vi "force_ctrl_test.vi"() -> ()   [LabVIEW 2014]
uses:
  <vilib>/eio/EIONode/EIONode.xnode
  <vilib>/rvi/FXPMathLib/FxpMul/XNode/nifxpmath_Multiplier.xnode
  <vilib>/rvi/FXPMathLib/sim/FxpSim.dll
  <vilib>/rvi/eio/common/nirviEmuTemplateMethod_errors.vi
  <vilib>/rvi/FXPMathLib/FxpSinAndCos/XNode/nifxpmath_SinAndCos.xnode
  <vilib>/rvi/FXPMathLib/FxpSinAndCos/simVIs/DllFxpSinAndCosTemp_sub.vi
  <vilib>/rvi/FXPMathLib/FxpSinAndCos/subVIs/nifxpmath_SinAndCos_SimConfig.ctl
  <vilib>/rvi/Analysis/measure/butterworth/XNode/niFpgaButterworthFilter.xnode
  <vilib>/rvi/FXPMathLib/FxpSub/XNode/nifxpmath_Sub.xnode
  <vilib>/rvi/FXPMathLib/FxpAdd/XNode/nifxpmath_Add.xnode
  <vilib>/rvi/DataTransferAndStorage/Container/XNode/niFpgaContainer.xnode
  <vilib>/rvi/interface/RandomDataEmulation/nirviRandomDataFpgaMultiElementTemplate.vi
panel:
  out "Mod6/AI0":fxp<+/-,24,-4>
  out "Chirp Frequency (Hz)":fxp<+/-,30,7>
  in  "Frequency_start (Hz)":fxp<+/-,36,4>
  in  "Target time (s)":fxp<+/-,36,11>
  in  "Frequency_end (Hz)":fxp<+/-,33,6>
  out "Chirp_signal":fxp<+/-,36,11>
  in  "Sin wave ampitude (mm)":fxp<+/-,33,6>
  out "omega (M_avg)":fxp<+/-,64,35>
  out "D_d (M_avg)":fxp<+/-,64,32>
  in  "D_d_M_avg_Tc (uSec)":u32
  out "omega (M)":fxp<+/-,64,30>
  out "D_d (M)":fxp<+/-,64,27>
  in  "D_d_M_Tc (uSec)":u32 format="%#_6f"
  out "D_d (T)":fxp<+/-,46,10>
  out "omega(T)":fxp<+/-,20,9>
  in  "Velocity Estimation":i16(ring) items=["M_avg method", "M method", "T method"]
  out "Dr_ramp":fxp<+/-,64,30>
  out "Dr_slope":fxp<+/-,33,17>
  in  "Dr_time":fxp<+/-,16,11>
  out "Dr_sin":fxp<+/-,28,11>
  out "Dr_sin_d":fxp<+/-,64,16>
  out "Dr_sin_dd":fxp<+/-,64,25>
  out "Sin omega":fxp<+/-,41,8>
  in  "Sin offset":fxp<+/-,27,10>
  in  "Sin magnitude":fxp<+/-,11,8>
  in  "Sin wave frequency (Hz)":fxp<+/-,21,5>
  out "Time now (s)":fxp<+,52,14>
  out "Dr":fxp<+/-,64,31>
  in  "Dr_end":fxp<+/-,16,11>
  in  "Command type":i16(ring) items=["Step", "Ramp", "Sine", "Chirp"]
  out "D_i":fxp<+/-,38,10>
  in  "D_tolorence":fxp<+/-,27,3>
  in  "Ki":fxp<+/-,36,10>
  out "D_error":fxp<+/-,36,10>
  in  "Direction":bool
  out "Fmr_PD":fxp<+/-,36,10>
  in  "Kd":fxp<+/-,36,10>
  in  "Kp":fxp<+/-,33,10>
  in  "scaled coefficients_D_dd":i32[](array[numeric])=[780119100, 146811362]
  out "D_dd":fxp<+/-,36,29>
  in  "Ini coe.":bool
  out "va":fxp<+/-,43,8>
  out "vb":fxp<+/-,43,8>
  in  "stop motor":bool
  out "vq_F":fxp<+/-,25,5> format="%.57g"
  out "vd_F":fxp<+/-,25,5>
  out "D_d (mm/s)":fxp<+/-,32,12>
  out "mt":u32
  out "omega (rad/s)":fxp<+/-,36,10>
  in  "mt0":u32
  out "D(mm)":fxp<+/-,33,10>
  out "rad(NrTheta)":fxp<+/-,33,10>
  out "Encoder Position":i32
  in  "Encoder Reset":bool
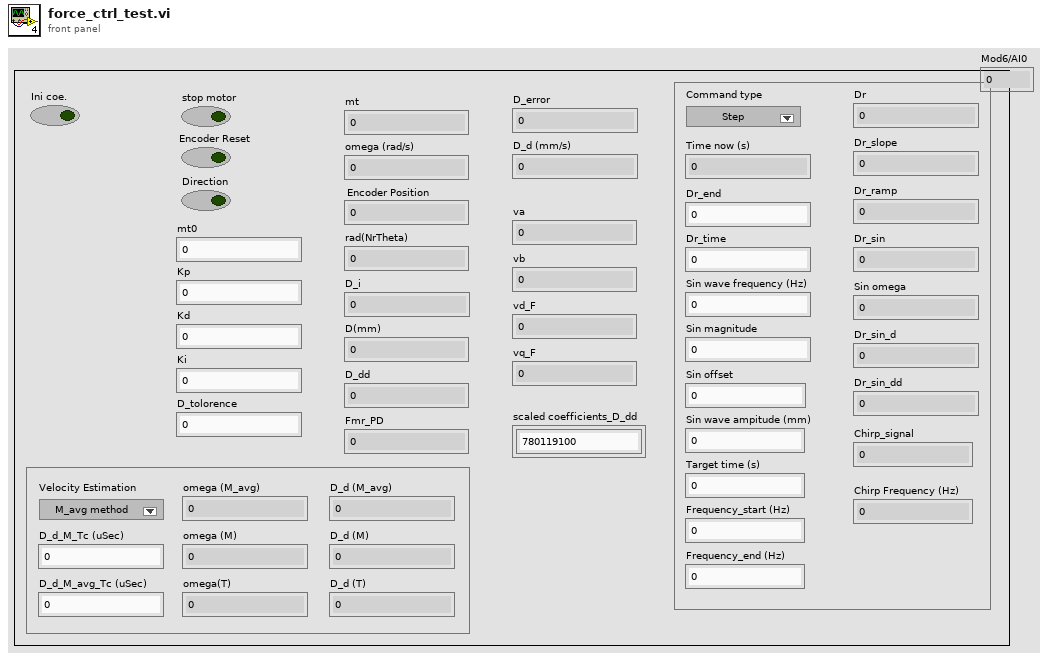
[diagram p1: front panel]
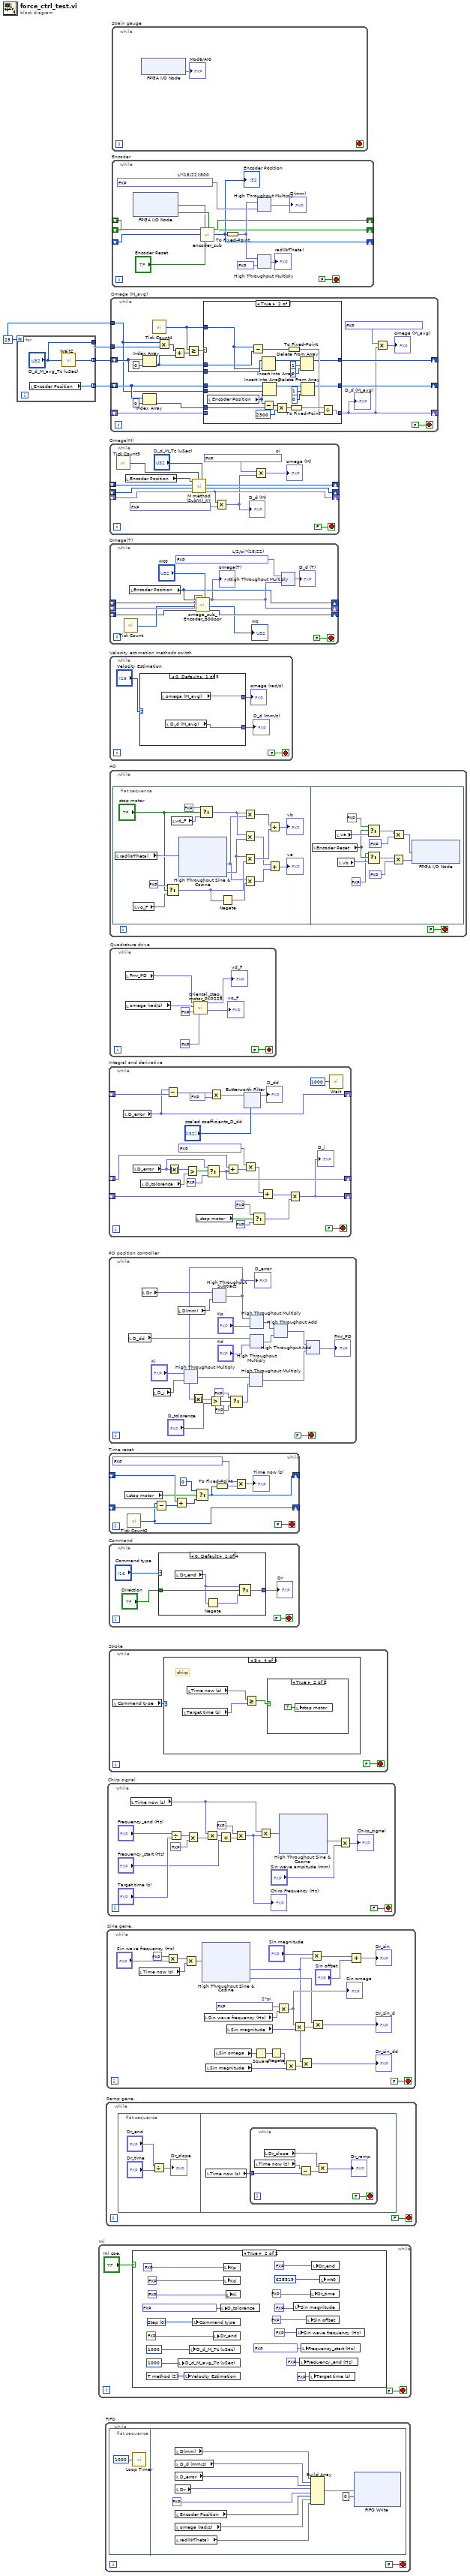
[diagram p0: block diagram]
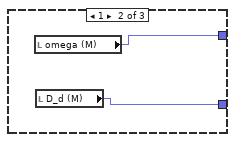
[diagram p3: hidden frame]
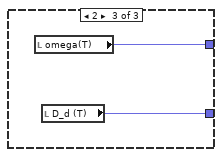
[diagram p4: hidden frame]
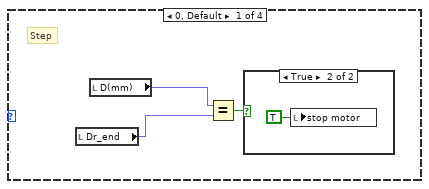
[diagram p5: hidden frame]
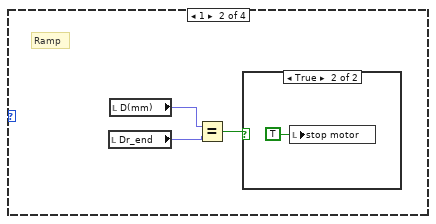
[diagram p7: hidden frame]
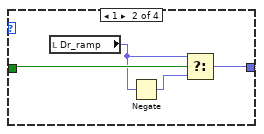
[diagram p11: hidden frame]
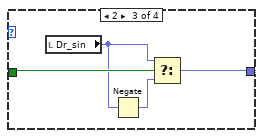
[diagram p12: hidden frame]
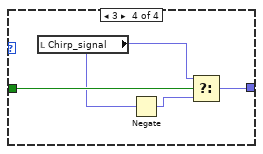
[diagram p13: hidden frame]
diagram:
  w4 = 25
  n1 = for {
    N: w4 -> [_]
    tunnel: ["D_d_M_avg_Tc (uSec)"] -> w1
    tunnel: [w6] -> w3 mode=indexing
    tunnel: [w5] -> w2 mode=indexing
    n2 = local read "Encoder Position"() -> (w5:i32)
    n3 = call "Wait2"("Count(uSec)"="D_d_M_avg_Tc (uSec)") -> ("Tick Count(uSec)"=w6:u32)
  }
  n4 = while "Ini" {
    stop <- FALSE stop-if-true
    n5 = case shown="True" "Ini coe." {
      frame False {
      }
      frame True {
        w12 = i16 0 items=["Step", "Ramp", "Sine", "Chirp"] ("Command type")
        w15 = i16 2 items=["M_avg method", "M method", "T method"] ("Velocity Estimation")
        n6 = local write "D_d_M_avg_Tc (uSec)"(u32 1000 ("D_d_M_avg_Tc (uSec)")) -> ()
        n7 = local write "Velocity Estimation"(w15) -> ()
        n8 = local write "D_d_M_Tc (uSec)"(u32 1000 ("D_d_M_Tc (uSec)")) -> ()
        n9 = local write "Command type"(w12) -> ()
        n10 = local write "Dr_end"(fxp<+/-,16,11> 20.0 ("Dr_end")) -> ()
        n11 = local write "D_tolorence"(fxp<+/-,27,3> 0.009999990463256836 ("D_tolorence")) -> ()
        n12 = local write "Kp"(fxp<+/-,20,12> 30.0 ("Kp")) -> ()
        n13 = local write "Kd"(fxp<+/-,20,8> 0.0 ("Kd")) -> ()
        n14 = local write "Ki"(fxp<+/-,20,6> 0.0 ("D_i")) -> ()
        n15 = local write "Sin magnitude"(fxp<+/-,11,8> 20.0 ("Sin magnitude")) -> ()
        n16 = local write "Sin wave frequency (Hz)"(fxp<+/-,21,5> 0.5 ("Sin wave frequency (Hz)")) -> ()
        n17 = local write "Frequency_end (Hz)"(fxp<+/-,23,8> 10.0 ("Frequency_end (Hz)")) -> ()
        n18 = local write "Frequency_start (Hz)"(fxp<+/-,20,5> 0.010009765625 ("Frequency_start (Hz)")) -> ()
        n19 = local write "Sin offset"(fxp<+/-,27,10> 0.0 ("Sin offset")) -> ()
        n20 = local write "Target time (s)"(fxp<+/-,24,9> 60.0 ("Target time (s)")) -> ()
        n21 = local write "Dr_time"(fxp<+/-,16,11> 5.0 ("Dr_time")) -> ()
        n22 = local write "Dr_end"(fxp<+/-,11,7> 20.0 ("Fmr")) -> ()
        n23 = local write "mt0"(u32 628319 ("mt0")) -> ()
      }
    }
  }
  n24 = while "FIFO" {
    stop <- FALSE stop-if-true
    n25 = flat-sequence {
      frame #0 {
        n26 = call "Loop Timer"("Count(uSec)"=u32 1000) -> ()  [unwired: 1 out]
      }
      frame #1 {
        n27 = local read "D(mm)"() -> (w37:fxp<+/-,33,10>)
        n28 = local read "D_d (mm/s)"() -> (w36:fxp<+/-,32,12>)
        n29 = local read "D_error"() -> (w35:fxp<+/-,36,10>)
        n30 = local read "Dr"() -> (w34:fxp<+/-,64,31>)
        n31 = local read "Encoder Position"() -> (w33:i32)
        n32 = local read "omega (rad/s)"() -> (w32:fxp<+/-,36,10>)
        n33 = local read "rad(NrTheta)"() -> (w31:fxp<+/-,33,10>)
        n34 = Build Array(w37, w36, w35, w34, fxp<+/-,64,32> 0.0 ("element"), w33, w32, w31) -> (w38:fxp<+/-,64,32>[])
        n35 = xnode ("FIFO Write")("Element"=w38, "Timeout"=0) -> ()  [unwired: 1 in, 2 out]
      }
    }
  }
  n36 = while "Ramp gene." {
    stop <- FALSE stop-if-true
    n37 = flat-sequence {
      frame #0 {
        n38 = Divide(x="Dr_end", y="Dr_time") -> (x/y=→"Dr_slope":fxp<+/-,33,17>)
      }
      frame #1 {
        n39 = local read "Time now (s)"() -> (w44:fxp<+,52,14>)
        n40 = while {
          tunnel: w44 -> [w50]
          stop <- FALSE stop-if-true
          n41 = local read "Time now (s)"() -> (w47:fxp<+,52,14>)
          n42 = local read "Dr_slope"() -> (w48:fxp<+/-,33,17>)
          n43 = Subtract(x=w47, y=w50) -> (x-y=w49:fxp<+/-,53,15>)
          n44 = Multiply(x=w48, y=w49) -> (x*y=→"Dr_ramp":fxp<+/-,64,30>)
        }
      }
    }
  }
  n45 = while "Sine gene." {
    stop <- FALSE stop-if-true
    w68 = fxp<+,20,3> 6.2831878662109375  # 2*pi
    n46 = local read "Time now (s)"() -> (w71:fxp<+,52,14>)
    n47 = Multiply(x=fxp<+,1,2> 2.0, y="Sin wave frequency (Hz)") -> (x*y=w72:fxp<+/-,21,6>)
    n48 = Multiply(x=w72, y=w71) -> (x*y=w52:fxp<+/-,64,20>)
    n49 = xnode "High Throughput Sine & Cosine"("x (pi)"=w52) -> ("sin(x)"=w56:fxp<+/-,16,2>, "cos(x)"=w63:fxp<+/-,16,2>)
    n50 = local read "Sin wave frequency (Hz)"() -> (w67:fxp<+/-,21,5>)
    n51 = local read "Sin magnitude"() -> (w58:fxp<+/-,11,8>)
    n52 = local read "Sin omega"() -> (w59:fxp<+/-,41,8>)
    n53 = local read "Sin magnitude"() -> (w62:fxp<+/-,11,8>)
    n54 = Square(x=w59) -> (x^2=w60:fxp<+,64,14>)
    n55 = Negate(x=w60) -> (-x=w57:fxp<+/-,64,15>)
    n56 = Multiply(x=w68, y=w67) -> (x*y=w64:fxp<+/-,41,8>)
    "Sin omega" <- w64
    n57 = Multiply(x=w57, y=w58) -> (x*y=w61:fxp<+/-,64,23>)
    n58 = Multiply(x=w64, y=w62) -> (x*y=w69:fxp<+/-,51,15>)
    n59 = Multiply(x=w56, y=w61) -> (x*y=→"Dr_sin_dd":fxp<+/-,64,25>)
    n60 = Multiply(x="Sin magnitude", y=w56) -> (x*y=w70:fxp<+/-,27,10>)
    n61 = Multiply(x=w63, y=w69) -> (x*y=→"Dr_sin_d":fxp<+/-,64,16>)
    n62 = Add(x=w70, y="Sin offset") -> (x+y=→"Dr_sin":fxp<+/-,28,11>)
  }
  n63 = while "Chirp signal" {
    stop <- FALSE stop-if-true
    n64 = local read "Time now (s)"() -> (w111:fxp<+,52,14>)
    n65 = Divide(x="Frequency_end (Hz)", y="Target time (s)") -> (x/y=w114:fxp<+/-,24,8>)
    n66 = Multiply(x=w114, y=fxp<+/-,24,9> 0.5) -> (x*y=w112:fxp<+/-,33,8>)
    n67 = Multiply(x=w111, y=w112) -> (x*y=w110:fxp<+/-,36,12>)
    n68 = Add(x=w110, y="Frequency_start (Hz)") -> (x+y=w106:fxp<+/-,38,13>)
    n69 = Multiply(x=fxp<+/-,3,3> 2.0, y=w106) -> (x*y=w105:fxp<+/-,38,13>)
    "Chirp Frequency (Hz)" <- w105
    n70 = Multiply(x=w111, y=w105) -> (x*y=w117:fxp<+/-,39,16>)
    n71 = xnode "High Throughput Sine & Cosine"("x (pi)"=w117) -> ("sin(x)"=w120:fxp<+/-,16,2>)  [unwired: 1 out]
    n72 = Multiply(x=w120, y="Sin wave ampitude (mm)") -> (x*y=→"Chirp_signal":fxp<+/-,36,11>)
  }
  n73 = while "Integral and derivative" {
    shift-right: [w151] -> _
    shift-left: _ -> [w175]
    shift-right: [w162] -> _
    shift-left: _ -> [w163]
    shift-right: [w152] -> _
    shift-left: _ -> [w156]
    stop <- FALSE stop-if-true
    n74 = local read "D_error"() -> (w151:fxp<+/-,36,10>)
    n75 = local read "D_error"() -> (w164:fxp<+/-,36,10>)
    n76 = local read "D_tolorence"() -> (w167:fxp<+/-,27,3>)
    n77 = Subtract(x=w151, y=w175) -> (x-y=w174:fxp<+/-,37,11>)
    n78 = Absolute Value(x=w164) -> (abs(x)=w168:fxp<+,36,10>)
    n79 = Greater?(x=w168, y=w167) -> (0:w166:bool)
    n80 = local read "stop motor"() -> (w159:bool)
    n81 = Select(t=w164, s=w166, f=fxp<+,24,11> 0.0) -> (s? t:f=w162:fxp<+/-,38,12>)
    n82 = Multiply(x=w174, y=fxp<+/-,33,13> 1000.0) -> (x*y=w172:fxp<+/-,64,23>)
    n83 = Add(x=w163, y=w162) -> (x+y=w161:fxp<+/-,39,10>)
    n84 = Multiply(x=fxp<+/-,30,12> 0.000499725341796875, y=w161) -> (x*y=w155:fxp<+/-,39,10>)
    n85 = xnode "Butterworth Filter"("input data"=w172, "scaled coefficients"="scaled coefficients_D_dd") -> ("output data"=→"D_dd":fxp<+/-,36,27>)  [unwired: 1 in]
    n86 = Select(t=fxp<+,1,1> 0.0, s=w159, f=fxp<+,1,1> 1.0) -> (s? t:f=w153:fxp<+,1,1>)
    n87 = Add(x=w155, y=w156) -> (x+y=w154:fxp<+/-,36,10>)
    n88 = Multiply(x=w154, y=w153) -> (x*y=w152:fxp<+/-,36,10>)
    "D_i" <- w152
    n89 = call "Wait"("Count(uSec)"=u32 1000) -> ()  [unwired: 1 out]
  }
  n90 = while "PD position controller" {
    stop <- FALSE stop-if-true
    n91 = local read "D_dd"() -> (w201:fxp<+/-,36,29>)
    n92 = local read "Dr"() -> (w185:fxp<+/-,64,31>)
    n93 = local read "D_i"() -> (w196:fxp<+/-,38,10>)
    n94 = local read "D(mm)"() -> (w205:fxp<+/-,33,10>)
    n95 = xnode ("High Throughput Multiply")("x"="Ki", "y"=w196) -> ("x*y"=w190:fxp<+/-,64,20>)
    n96 = xnode "High Throughput Subtract"("x"=w185, "y"=w205) -> ("x-y"=w194:fxp<+/-,64,32>)
    "D_error" <- w194
    n97 = Absolute Value(x=w194) -> (abs(x)=w195:fxp<+,64,32>)
    n98 = Greater?(x=w195, y="D_tolorence") -> (0:w193:bool)
    n99 = Select(t=fxp<+,10,2> 1.0, s=w193, f=fxp<+,10,2> 0.0) -> (s? t:f=w189:fxp<+,10,2>)
    n100 = xnode ("High Throughput Multiply")("x"=w190, "y"=w189) -> ("x*y"=w186:fxp<+/-,64,22>)
    n101 = xnode ("High Throughput Multiply")("x"=w194, "y"="Kp") -> ("x*y"=w203:fxp<+/-,64,42>)
    n102 = xnode ("High Throughput Multiply")("x"=w201, "y"="Kd") -> ("x*y"=w202:fxp<+/-,64,39>)
    n103 = xnode ("High Throughput Add")("x"=w203, "y"=w202) -> ("x+y"=w187:fxp<+/-,64,43>)
    n104 = xnode ("High Throughput Add")("x"=w187, "y"=w186) -> ("x+y"=→"Fmr_PD":fxp<+/-,64,44>)
  }
  n105 = while "Time reset" {
    shift-right: [w209] -> _
    shift-left: _ -> [w216]
    shift-right: [w211] -> _
    shift-left: _ -> [w212]
    stop <- FALSE stop-if-true
    n106 = local read "stop motor"() -> (w214:bool)
    n107 = call "Tick Count2"() -> ("Tick Count(uSec)"=w211:u32)
    n108 = Subtract(x=w211, y=w212) -> (x-y=w217:u32)
    n109 = Add(x=w216, y=w217) -> (x+y=w215:u32)
    n110 = Select(t=u32 0, s=w214, f=w215) -> (s? t:f=w209:u32)
    n111 = To Fixed-Point(number=w209) -> (fixed-point=w208:fxp<+,32,32>)  [unwired: 1 in]
    n112 = Multiply(x=fxp<+,20,-18> 1.0000003385357559e-06, y=w208) -> (x*y=→"Time now (s)":fxp<+,52,14>)
  }
  n113 = while "Stroke" {
    stop <- FALSE stop-if-true
    n114 = local read "Command type"() -> (w219:i16)
    n115 = case shown="3" w219 {
      frame 0, Default {
        # "Step"
        n116 = local read "Dr_end"() -> (w220:fxp<+/-,16,11>)
        n117 = local read "D(mm)"() -> (w221:fxp<+/-,33,10>)
        n118 = Equal?(x=w221, y=w220) -> (x = y?=w222:bool)
        n119 = case shown="True" w222 {
          frame False {
          }
          frame True {
            n120 = local write "stop motor"(TRUE ("stop motor")) -> ()
          }
        }
      }
      frame 1 {
        # "Ramp"
        n121 = local read "Dr_end"() -> (w226:fxp<+/-,16,11>)
        n122 = local read "D(mm)"() -> (w224:fxp<+/-,33,10>)
        n123 = Equal?(x=w224, y=w226) -> (x = y?=w225:bool)
        n124 = case shown="True" w225 {
          frame False {
          }
          frame True {
            n125 = local write "stop motor"(TRUE ("stop motor")) -> ()
          }
        }
      }
      frame 2 {
      }
      frame 3 {
        # "chirp"
        n126 = local read "Target time (s)"() -> (w229:fxp<+/-,36,11>)
        n127 = local read "Time now (s)"() -> (w228:fxp<+,52,14>)
        n128 = Greater Or Equal?(x=w228, y=w229) -> (x >= y?=w230:bool)
        n129 = case shown="True" w230 {
          frame False {
          }
          frame True {
            n130 = local write "stop motor"(TRUE ("stop motor")) -> ()
          }
        }
      }
    }
  }
  n131 = while "Command" {
    stop <- FALSE stop-if-true
    n132 = case shown="0, Default" "Command type" {
      tunnel: [w236 w240 w244 w248] -> w234
      tunnel: "Direction" -> [w239 w243 w247 w251]
      frame 0, Default {
        n133 = local read "Dr_end"() -> (w238:fxp<+/-,16,11>)
        n134 = Negate(x=w238) -> (-x=w237:fxp<+/-,17,12>)
        n135 = Select(t=w238, s=w239, f=w237) -> (s? t:f=w236:fxp<+/-,17,12>)
      }
      frame 1 {
        n136 = local read "Dr_ramp"() -> (w241:fxp<+/-,64,30>)
        n137 = Negate(x=w241) -> (-x=w242:fxp<+/-,64,31>)
        n138 = Select(t=w241, s=w243, f=w242) -> (s? t:f=w240:fxp<+/-,64,31>)
      }
      frame 2 {
        n139 = local read "Dr_sin"() -> (w245:fxp<+/-,28,11>)
        n140 = Negate(x=w245) -> (-x=w246:fxp<+/-,27,10>)
        n141 = Select(t=w245, s=w247, f=w246) -> (s? t:f=w244:fxp<+/-,28,11>)
      }
      frame 3 {
        n142 = local read "Chirp_signal"() -> (w249:fxp<+/-,36,11>)
        n143 = Negate(x=w249) -> (-x=w250:fxp<+/-,37,12>)
        n144 = Select(t=w249, s=w251, f=w250) -> (s? t:f=w248:fxp<+/-,37,12>)
      }
    }
    "Dr" <- w234
  }
  n145 = while "Omega(M)" {
    shift-right: [w263] -> _
    shift-left: _ -> [w264]
    shift-right: [w259] -> _
    shift-left: _ -> [w260]
    shift-right: [w257] -> _
    shift-left: _ -> [w258]
    stop <- FALSE stop-if-true
    w254 = fxp<+/-,27,3> 3.1415926218032837  # pi
    n146 = call "Tick Count3"() -> ("Tick Count(mSec)"=w262:u32)
    n147 = local read "Encoder Position"() -> (w265:i32)
    n148 = call "M method (SubVI)_KY.vi"("Tc (mSec)"="D_d_M_Tc (uSec)", "Tick Count (mSec)"=w262, "Encoder velocity_pre (pulse/s)"=w258, "Shift Register in 2"=w260, "Shift Register in 1"=w264, "Encoder pulses"=w265) -> ("Encoder velocity (pulse/s)"=w257:fxp<+/-,64,32>, "Shift Register out 2"=w259:i32, "Shift Register out 1"=w263:u32)  [unwired: 3 in]
    n149 = Multiply(x=w257, y=fxp<+/-,20,-5> 0.002499997615814209) -> (x*y=w255:fxp<+/-,64,27>)
    "D_d (M)" <- w255
    n150 = Multiply(x=w254, y=w255) -> (x*y=→"omega (M)":fxp<+/-,64,30>)
  }
  n151 = while "Omega(T)" {
    shift-right: [w275] -> _
    shift-left: _ -> [w276]
    shift-right: [w268] -> _
    shift-left: _ -> [w274]
    shift-right: [w271] -> _
    shift-left: _ -> [w272]
    stop <- FALSE stop-if-true
    w269 = fxp<+/-,32,0> 0.2604353614151478  # L/2/pi*(18/22)
    n152 = call "Tick Count"() -> ("Tick Count(Ticks)"=w273:u32)
    n153 = local read "Encoder Position"() -> (w275:i32)
    n154 = call "omega_sub_Encoder_800ppr.vi"("mt0"="mt0", "omega_pre"=w274, "ticks_m_pre"=w272, "ticks"=w273, "count_pre"=w276, "count"=w275) -> ("ticks_m"=w271:u32, "mt"=→"mt":u32, "omega"=w268:fxp<+/-,20,9>)  [unwired: 3 in]
    "omega(T)" <- w268
    n155 = xnode ("High Throughput Multiply")("x"=w269, "y"=w268) -> ("x*y"=→"D_d (T)":fxp<+/-,52,9>)
  }
  n156 = while "Velocity estimation methods switch" {
    stop <- FALSE stop-if-true
    n157 = case shown="0, Default" "Velocity Estimation" {
      tunnel: [w283 w285 w287] -> w280
      tunnel: [w282 w284 w286] -> w279
      frame 0, Default {
        n158 = local read "omega (M_avg)"() -> (w283:fxp<+/-,64,35>)
        n159 = local read "D_d (M_avg)"() -> (w282:fxp<+/-,64,32>)
      }
      frame 1 {
        n160 = local read "omega (M)"() -> (w285:fxp<+/-,64,30>)
        n161 = local read "D_d (M)"() -> (w284:fxp<+/-,64,27>)
      }
      frame 2 {
        n162 = local read "omega(T)"() -> (w287:fxp<+/-,20,9>)
        n163 = local read "D_d (T)"() -> (w286:fxp<+/-,46,10>)
      }
    }
    "D_d (mm/s)" <- w279
    "omega (rad/s)" <- w280
  }
  n164 = while "AO" {
    stop <- FALSE stop-if-true
    n165 = flat-sequence {
      frame #0 {
        n166 = local read "rad(NrTheta)"() -> (w304:fxp<+/-,33,10>)
        n167 = local read "vq_F"() -> (w302:fxp<+/-,25,5>)
        n168 = Select(t=fxp<+,20,5> 0.0, s="stop motor", f=w302) -> (s? t:f=w299:fxp<+/-,26,6>)
        n169 = local read "vd_F"() -> (w303:fxp<+/-,25,5>)
        n170 = xnode "High Throughput Sine & Cosine"("x (pi)"=w304) -> ("sin(x)"=w295:fxp<+/-,17,2>, "cos(x)"=w297:fxp<+/-,17,2>)
        n171 = Select(t=fxp<+,20,5> 0.0, s="stop motor", f=w303) -> (s? t:f=w296:fxp<+/-,26,6>)
        n172 = Negate(x=w299) -> (-x=w298:fxp<+/-,26,6>)
        n173 = Multiply(x=w296, y=w295) -> (x*y=w294:fxp<+/-,42,7>)
        n174 = Multiply(x=w296, y=w297) -> (x*y=w292:fxp<+/-,42,7>)
        n175 = Multiply(x=w297, y=w299) -> (x*y=w293:fxp<+/-,42,7>)
        n176 = Multiply(x=w295, y=w298) -> (x*y=w291:fxp<+/-,42,7>)
        n177 = Add(x=w294, y=w293) -> (x+y=→"vb":fxp<+/-,43,8>)
        n178 = Add(x=w292, y=w291) -> (x+y=→"va":fxp<+/-,43,8>)
      }
      frame #1 {
        n179 = local read "Encoder Reset"() -> (w338:bool)
        n180 = local read "va"() -> (w340:fxp<+/-,43,8>)
        n181 = local read "vb"() -> (w339:fxp<+/-,43,8>)
        n182 = Select(t=fxp<+/-,20,5> 3.0 ("y"), s=w338, f=w340) -> (s? t:f=w341:fxp<+/-,43,8>)
        n183 = Select(t=fxp<+/-,20,5> 0.0 ("y"), s=w338, f=w339) -> (s? t:f=w342:fxp<+/-,43,8>)
        n184 = Multiply(x=w342, y=fxp<+/-,20,5> -0.5) -> (x*y=w346:fxp<+/-,62,12>)
        n185 = Multiply(x=w341, y=fxp<+/-,20,5> -0.5) -> (x*y=w345:fxp<+/-,62,12>)
        n186 = xnode "FPGA I/O Node"("Mod8/AO2"=w345, "Mod8/AO3"=w346) -> ()  [unwired: 2 in, 2 out]
      }
    }
  }
  n187 = while "Quadrature drive" {
    stop <- FALSE stop-if-true
    n188 = local read "Fmr_PD"() -> (w347:fxp<+/-,36,10>)
    n189 = local read "omega (rad/s)"() -> (w349:fxp<+/-,36,10>)
    n190 = call "Oriental_step_motor_PKP225.vi"("F_Threshold"=fxp<+,12,12> 10.0, "dFmr"=fxp<+/-,25,15> 0.0, "omega"=w349, "Fmr"=w347) -> ("vq_F"=→"vq_F":fxp<+/-,20,5>, "vd_F"=→"vd_F":fxp<+/-,20,5>)  [unwired: 6 in]
  }
  n191 = while "Omega (M_avg)" {
    tunnel: w4 -> [w365]
    shift-right: [w358] -> _
    shift-left: w3 -> [w369]
    shift-right: [w357] -> _
    shift-left: _ -> [w360]
    shift-right: [w359] -> _
    shift-left: w2 -> [w368]
    tunnel: w1 -> [w362]
    stop <- FALSE stop-if-true
    n192 = Index Array(array=w369, index=0) -> (element=w363:u32)
    n193 = Index Array(array=w368, index=0) -> (element=w364:i32)
    n194 = call "Tick Count4"() -> ("Tick Count(uSec)"=w366:u32)
    n195 = Multiply(x=w365, y=w362) -> (x*y=w370:u32)
    n196 = Add(x=w370, y=w363) -> (x+y=w367:u32)
    n197 = Greater Or Equal?(x=w366, y=w367) -> (x >= y?=w361:bool)
    n198 = case shown="True" w361 {
      tunnel: w369 -> [w375 w392]
      tunnel: w368 -> [w374 w391]
      tunnel: w366 -> [_ w384]
      tunnel: w365 -> [_ w390]
      tunnel: w364 -> [_ w388]
      tunnel: w363 -> [_ w383]
      tunnel: w360 -> [w373 _]
      tunnel: [w374 w378] -> w359
      tunnel: [w375 w377] -> w358
      tunnel: [w373 w376] -> w357
      frame False {
      }
      frame True {
        n199 = local read "Encoder Position"() -> (w389:i32)
        n200 = Subtract(x=w384, y=w383) -> (x-y=w381:u32)
        n201 = Insert Into Array(array=w392, new element=w384) -> (w393:u32[])  [unwired: 1 in]
        n202 = Subtract(x=w389, y=w388) -> (x-y=w387:i32)
        n203 = Insert Into Array(array=w391, index=w390, new element=w389) -> (w394:i32[])
        n204 = Multiply(x=w387, y=2500) -> (x*y=w385:i32)
        n205 = To Fixed-Point(number=w381) -> (fixed-point=w379:fxp<+,32,32>)  [unwired: 1 in]
        n206 = To Fixed-Point(number=w385) -> (fixed-point=w380:fxp<+/-,32,32>)  [unwired: 1 in]
        n207 = Delete From Array(array=w393, length=1, index=0) -> (array with subset deleted=w377:u32[])  [unwired: 1 out]
        n208 = Delete From Array(array=w394, length=1, index=0) -> (array with subset deleted=w378:i32[])  [unwired: 1 out]
        n209 = Divide(x=w380, y=w379) -> (x/y=w376:fxp<+/-,64,32>)
      }
    }
    "D_d (M_avg)" <- w357
    n210 = Multiply(x=fxp<+/-,27,3> 3.1415926218032837, y=w357) -> (x*y=→"omega (M_avg)":fxp<+/-,64,35>)
  }
  n211 = while "Strain gauge" {
    stop <- _ stop-if-true
    n212 = xnode "FPGA I/O Node"() -> ("Mod6/AI0"=→"Mod6/AI0":fxp<+/-,24,-4>)  [unwired: 1 in, 1 out]
  }
  n213 = while "Encoder" {
    shift-right: [w405] -> _
    shift-left: _ -> [w407]
    shift-right: [w404] -> _
    shift-left: _ -> [w406]
    shift-right: [w402] -> _
    shift-left: _ -> [w403]
    stop <- FALSE stop-if-true
    w409 = fxp<+/-,32,0> 0.0020454544574022293  # L*(18/22)/800
    n214 = xnode "FPGA I/O Node"() -> ("Mod4/DI3"=w412:bool, "Mod4/DI4"=w413:bool)  [unwired: 2 in, 2 out]
    n215 = call "encoder_sub.vi"("A_pre"=w407, "B_pre"=w406, "Encoder Position_pre"=w403, "A input"=w412, "Encoder Position Reset"="Encoder Reset", "B input"=w413) -> ("A"=w405:bool, "B"=w404:bool, "Encoder Position (Counts)"=w402:i32)  [unwired: 19 in]
    "Encoder Position" <- w402
    n216 = To Fixed-Point(number=w402) -> (fixed-point=w410:fxp<+/-,32,32>)  [unwired: 1 in]
    n217 = xnode ("High Throughput Multiply")("x"=w410, "y"=w409) -> ("x*y"=→"D(mm)":fxp<+/-,64,32>)
    n218 = xnode ("High Throughput Multiply")("x"=w410, "y"=fxp<+/-,24,0> 0.125) -> ("x*y"=→"rad(NrTheta)":fxp<+/-,56,32>)
  }
